vi "test ws standalone.vi"() -> ()   [LabVIEW 2016]
uses:
  http/websocket/standalone server/websocket connection parameters.ctl
  http/websocket/standalone server/websocket message type.ctl
  http/websocket/standalone server/websocket data packet.ctl
  http/websocket/standalone server/websocket standalone server.lvclass
panel:
  in  "send txt":bool
  in  "DATA to send":string
  out "conn idx":i32
  out "data":string
  out "message type":T1
  in  "parameters":T2={"port"=80, "supported subprotocols"=[]}
  in  "stop":bool
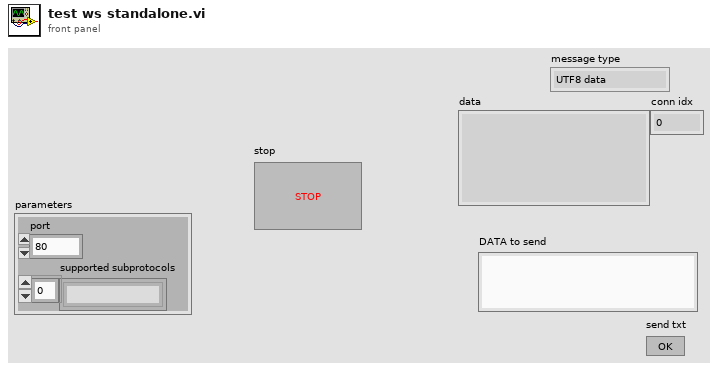
[diagram p1: front panel]
types:
  T1 = typedef "websocket standalone server.lvclass/websocket message type.ctl" = enum16{"UTF8 data", "binary data", "close", "ping", "pong"}
  T2 = typedef "websocket standalone server.lvclass/websocket connection parameters.ctl" = cluster{"port":u16, "supported subprotocols":string[]}
  T3 = typedef "websocket standalone server.lvclass/websocket data packet.ctl" = cluster{"message type":T1, "data":string}
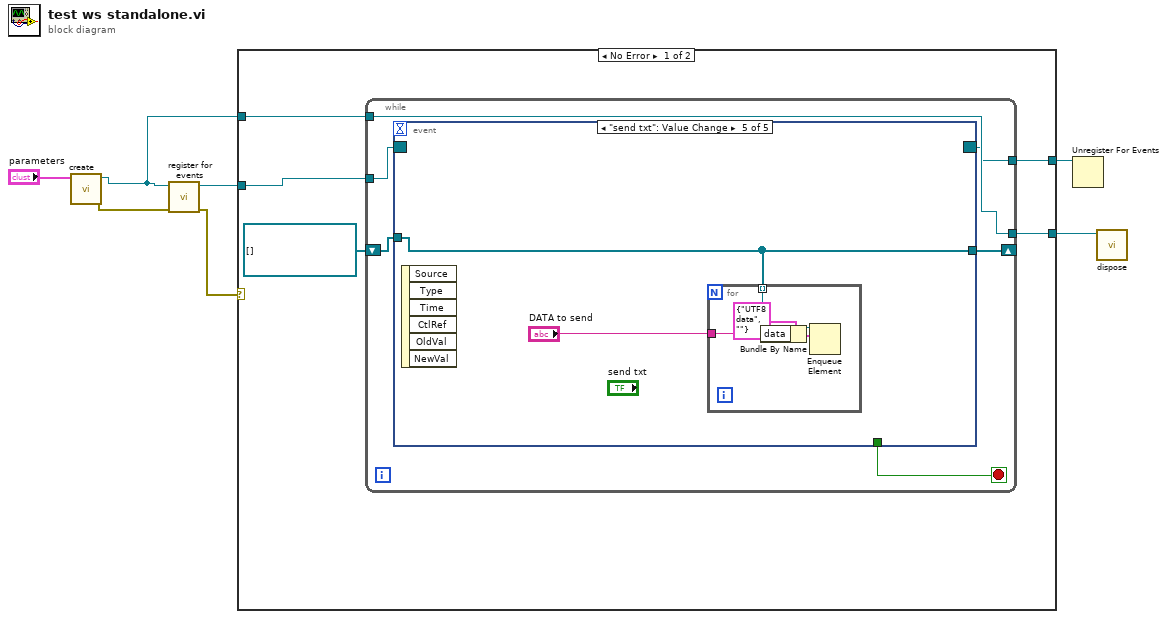
[diagram p0: block diagram]
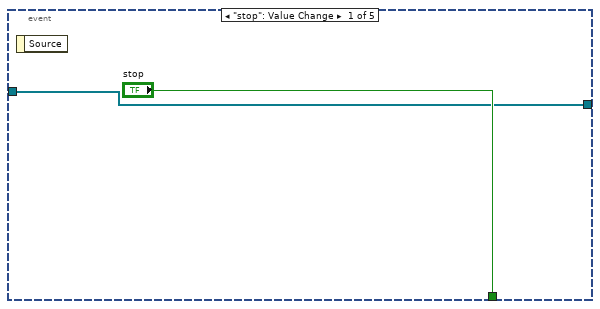
[diagram p2: hidden frame]
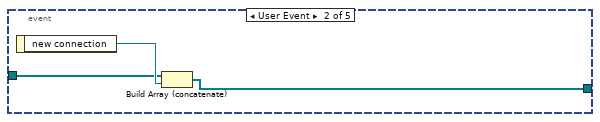
[diagram p3: hidden frame]
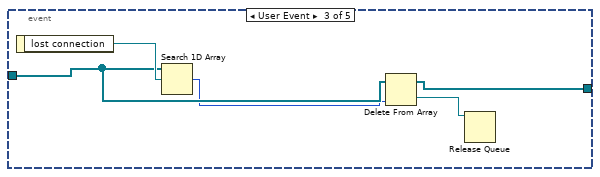
[diagram p4: hidden frame]
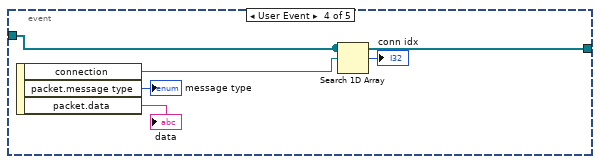
[diagram p5: hidden frame]
diagram:
  n1 = call "create.vi"("parameters"="parameters") -> ("error out"=w7:errorcluster, "websocket standalone server out"=w6:refnum<class "websocket standalone server.lvclass">)  [unwired: 9 in]
  n2 = call "register for events.vi"("error in"=w7, "websocket standalone server in"=w6) -> ("error out"=w1:errorcluster, "event registration"=w4:refnum<event-registration>)  [unwired: 8 in]
  n3 = case shown="No Error" w1 {
    tunnel: w6 -> [w12 w40]
    tunnel: [w11 w40] -> w5
    tunnel: w4 -> [w10 w41]
    tunnel: [w9 w41] -> w3
    frame No Error {
      n4 = while {
        tunnel: w12 -> [w17]
        tunnel: [w17] -> w11
        tunnel: w10 -> [w16]
        tunnel: [w15] -> w9
        shift-right: [w14] -> _
        shift-left: refnum<queue>[] [] -> [w13]
        stop <- w18 stop-if-true
        n5 = event shown="[4] \"send txt\": Value Change" {
          selector: w16 -> [_ _ _ _ _]
          dyn-events: [_ _ _ _ _] -> w15
          timeout: _ -> [_ _ _ _ _]
          tunnel: ["stop" _ _ _ _] -> w18
          tunnel: [w19 w22 w25 w31 w35] -> w14
          tunnel: w13 -> [w19 w21 w27 w31 w35]
          event "stop": Value Change {
            n6 = event-data() -> ()  [unwired: 1 in, 1 out]
          }
          event User Event {
            n7 = event-data() -> ("new connection"=w23:refnum<queue>)  [unwired: 1 in]
            n8 = Build Array (concatenate)(w21, w23) -> (w22:refnum<queue>[])
          }
          event User Event {
            n9 = event-data() -> ("lost connection"=w28:refnum<queue>)  [unwired: 1 in]
            n10 = Search 1D Array(1D array=w27, element=w28) -> (index of element=w26:i32)  [unwired: 1 in]
            n11 = Delete From Array(array=w27, index=w26) -> (deleted portion=w24:refnum<queue>, array with subset deleted=w25:refnum<queue>[])  [unwired: 1 in]
            n12 = Release Queue(queue=w24) -> ()  [unwired: 2 in, 3 out]
          }
          event User Event {
            n13 = event-data() -> ("connection"=w30:refnum<queue>, "packet.message type"=→"message type":T1, "packet.data"=→"data":string)  [unwired: 1 in]
            n14 = Search 1D Array(1D array=w31, element=w30) -> (index of element=→"conn idx":i32)  [unwired: 1 in]
          }
          event "send txt": Value Change {
            n15 = event-data() -> ()  [unwired: 1 in, 6 out]
            n16 = for {
              tunnel: w35 -> [w39] mode=indexing
              tunnel: "DATA to send" -> [w36]
              n17 = Bundle By Name(cluster=T3 {"message type"=enum."UTF8 data", "data"=""} ("element"), "data"=w36) -> (w37:T3)
              n18 = Enqueue Element(queue=w39, element=w37) -> ()  [unwired: 2 in, 3 out]
            }
          }
        }
      }
    }
    frame Error {
    }
  }
  n19 = Unregister For Events(event registration refnum=w3) -> ()  [unwired: 1 in, 1 out]
  n20 = call "dispose.vi"("websocket standalone server in"=w5) -> ()  [unwired: 10 in, 1 out]
